vi "Create Default Attributes.vi"(5 "Unique ID":string, 7 "Process Executive Ref":refnum<data-value>, 11 "Stop Pre-Soak in":refnum<class "Stop Pre-Soak.lvclass">) -> (3 "Stop Pre-Soak out":refnum<class "Stop Pre-Soak.lvclass">)   [LabVIEW 2019, in "Stop Pre-Soak.lvclass"]
uses:
  <vilib>/gpm_packages/@cs/Car-wash/Source/Process Steps/Stop Pre-Soak/Stop Pre-Soak.lvclass
  <vilib>/gpm_packages/@cs/test-executive/Source/Test Executive/ITestExecutive/ITest Executive.lvclass
  a9885f93-dc0e-4f0a-921f-571ad00b11c1.vi
  <vilib>/Utility/error.llb/Error Cluster From Error Code.vi
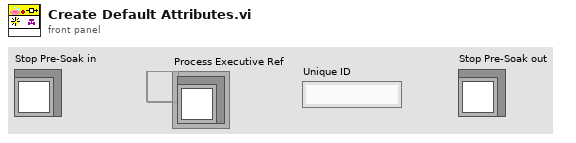
[diagram p1: front panel]
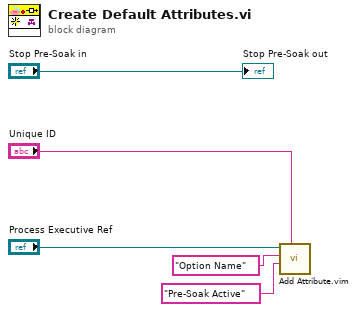
[diagram p0: block diagram]
diagram:
  n1 = call "Add Attribute.vim"("ID"="Unique ID", "Attribute"="Pre-Soak Active" ("Item Name"), "Attribute Name"="Option Name" ("Item Name"), "Test Executive Ref"="Process Executive Ref") -> ()  [unwired: 4 in, 4 out]
  "Stop Pre-Soak out" <- "Stop Pre-Soak in"
